vi "JoinFloatChannel.vi"(11 "Array":dbl[](array[numeric])) -> (3 "String":string)   [LabVIEW 2022 SP3]
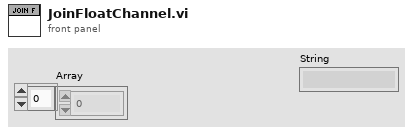
[diagram p1: front panel]
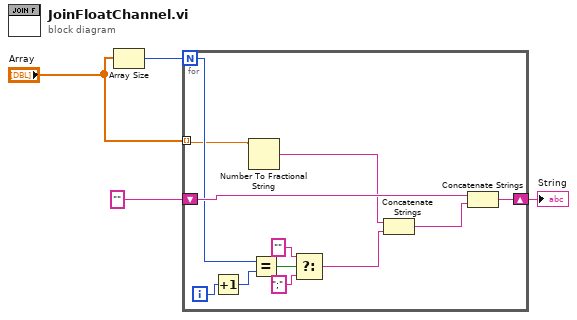
[diagram p0: block diagram]
diagram:
  n1 = Array Size(array="Array") -> (size(s)=w4:i32)
  n2 = for {
    N: w4 -> [w11]
    shift-right: [w16] -> w2
    shift-left: "" -> [w15]
    tunnel: "Array" -> [w6] mode=indexing
    i -> [w13]
    n3 = Increment(x=w13) -> (x+1=w12:i32)
    n4 = Number To Fractional String(number=w6) -> (F-format string=w5:string)  [unwired: 3 in]
    n5 = Equal?(x=w11, y=w12) -> (x = y?=w14:bool)
    n6 = Select(t="", s=w14, f=";") -> (s? t:f=w8:string)
    n7 = Concatenate Strings(w5, w8) -> (w7:string)
    n8 = Concatenate Strings(w15, w7) -> (w16:string)
  }
  "String" <- w2
